vi "Error Message.vi"(8 "firmware revision":string(combo), 11 "error number":i32) -> (2 "error message":string)   [LabVIEW 2020, in "Andeen-Hagerling 2700A.lvlib"]
doc: "This VI returns takes an error number and returns a text error message. Firmware version is a parameter also because error messages differ across firmware versions."
uses:
  Andeen-Hagerling 2700A.lvlib
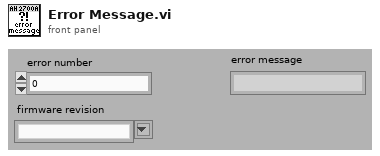
[diagram p1: front panel]
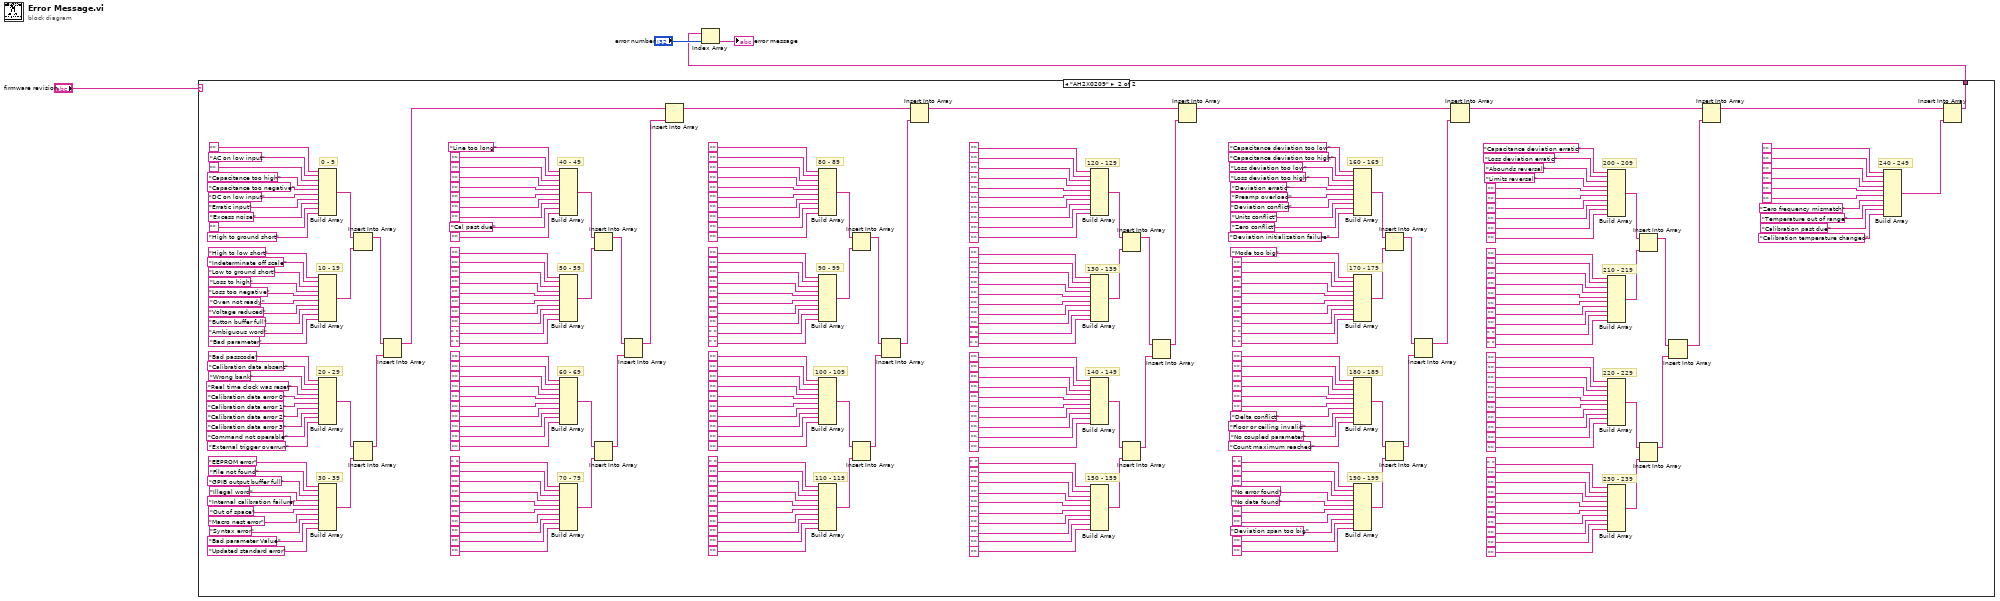
[diagram p0: block diagram]
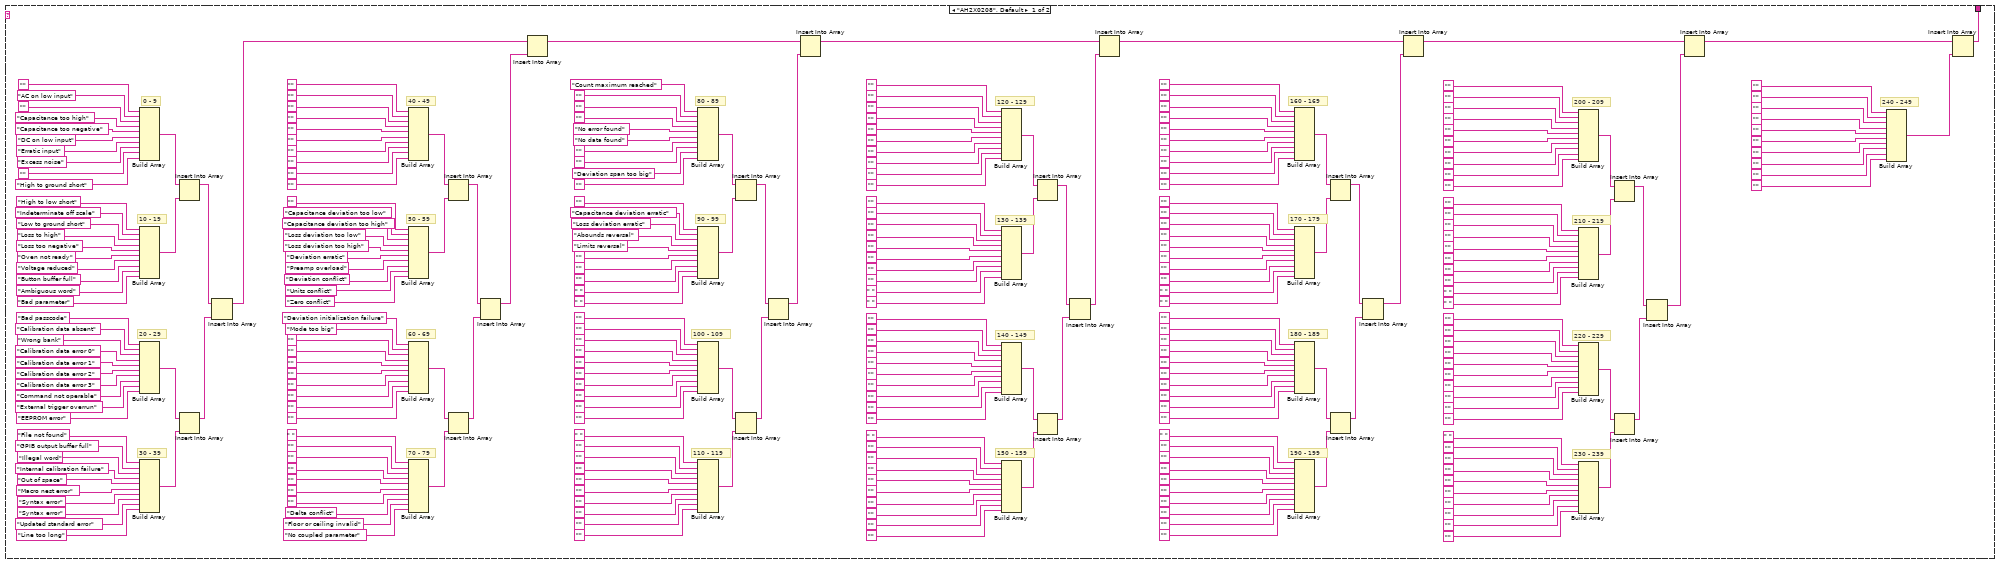
[diagram p2: hidden frame]
diagram:
  n1 = case shown="\"AH2X0209\"" "firmware revision" {
    tunnel: [w7 w304] -> w1
    frame "AH2X0208", Default {
      # "240 - 249"
      # "230 - 239"
      # "220 - 229"
      # "210 - 219"
      # "200 - 209"
      # "190 - 199"
      # "180 - 189"
      # "170 - 179"
      # "160 - 169"
      # "150 - 159"
      # "140 - 149"
      # "130 - 139"
      # "120 - 129"
      # "110 - 119"
      # "100 - 109"
      # "90 - 99"
      # "80 - 89"
      # "70 - 79"
      # "60 - 69"
      # "50 - 59"
      # "40 - 49"
      # "30 - 39"
      # "20 - 29"
      # "10 - 19"
      # "0 - 9"
      n2 = Build Array("", "AC on low input", "", "Capacitance too high", "Capacitance too negative", "DC on low input", "Erratic input", "Excess noise", "", "High to ground short") -> (w28:string[])
      n3 = Build Array("High to low short", "Indeterminate off scale", "Low to ground short", "Loss to high", "Loss too negative", "Oven not ready", "Voltage reduced", "Button buffer full", "Ambiguous word", "Bad parameter") -> (w29:string[])
      n4 = Build Array("Bad passcode", "Calibration data absent", "Wrong bank", "Calibration data error 0", "Calibration data error 1", "Calibration data error 2", "Calibration data error 3", "Command not operable", "External trigger overrun", "EEPROM error") -> (w40:string[])
      n5 = Build Array("File not found", "GPIB output buffer full", "Illegal word", "Internal calibration failure", "Out of space", "Macro nest error", "Syntax error", "Syntax error", "Updated standard error", "Line too long") -> (w41:string[])
      n6 = Insert Into Array(array=w28, new element=w29) -> (w52:string[])  [unwired: 1 in]
      n7 = Insert Into Array(array=w40, new element=w41) -> (w53:string[])  [unwired: 1 in]
      n8 = Insert Into Array(array=w52, new element=w53) -> (w292:string[])  [unwired: 1 in]
      n9 = Build Array("", "", "", "", "", "", "", "", "", "") -> (w72:string[])
      n10 = Build Array("", "Capacitance deviation too low", "Capacitance deviation too high", "Loss deviation too low", "Loss deviation too high", "Deviation erratic", "Preamp overload", "Deviation conflict", "Units conflict", "Zero conflict") -> (w73:string[])
      n11 = Build Array("Deviation initialization failure", "Mode too big", "", "", "", "", "", "", "", "") -> (w84:string[])
      n12 = Build Array(" ", "", "", "", "", "", "", "Delta conflict", "Floor or ceiling invalid", "No coupled parameter") -> (w85:string[])
      n13 = Insert Into Array(array=w72, new element=w73) -> (w96:string[])  [unwired: 1 in]
      n14 = Insert Into Array(array=w84, new element=w85) -> (w97:string[])  [unwired: 1 in]
      n15 = Insert Into Array(array=w96, new element=w97) -> (w293:string[])  [unwired: 1 in]
      n16 = Insert Into Array(array=w292, new element=w293) -> (w294:string[])  [unwired: 1 in]
      n17 = Build Array("Count maximum reached", "", "", "", "No error found", "No data found", "", "", "Deviation span too big", "") -> (w118:string[])
      n18 = Build Array("", "Capacitance deviation erratic", "Loss deviation erratic", "Abounds reversal", "Limits reversal", "", "", "", " ", " ") -> (w119:string[])
      n19 = Build Array("", "", "", "", "", "", "", "", "", "") -> (w130:string[])
      n20 = Build Array(" ", "", "", "", "", "", "", "", "", "") -> (w131:string[])
      n21 = Insert Into Array(array=w118, new element=w119) -> (w142:string[])  [unwired: 1 in]
      n22 = Insert Into Array(array=w130, new element=w131) -> (w143:string[])  [unwired: 1 in]
      n23 = Insert Into Array(array=w142, new element=w143) -> (w295:string[])  [unwired: 1 in]
      n24 = Insert Into Array(array=w294, new element=w295) -> (w296:string[])  [unwired: 1 in]
      n25 = Build Array("", "", "", "", "", "", "", "", "", "") -> (w164:string[])
      n26 = Build Array("", "", "", "", "", "", "", "", " ", " ") -> (w165:string[])
      n27 = Build Array("", "", "", "", "", "", "", "", "", "") -> (w176:string[])
      n28 = Build Array(" ", "", "", "", "", "", "", "", "", "") -> (w177:string[])
      n29 = Insert Into Array(array=w164, new element=w165) -> (w188:string[])  [unwired: 1 in]
      n30 = Insert Into Array(array=w176, new element=w177) -> (w189:string[])  [unwired: 1 in]
      n31 = Insert Into Array(array=w188, new element=w189) -> (w297:string[])  [unwired: 1 in]
      n32 = Insert Into Array(array=w296, new element=w297) -> (w298:string[])  [unwired: 1 in]
      n33 = Build Array("", "", "", "", "", "", "", "", "", "") -> (w210:string[])
      n34 = Build Array("", "", "", "", "", "", "", "", " ", " ") -> (w211:string[])
      n35 = Build Array("", "", "", "", "", "", "", "", "", "") -> (w222:string[])
      n36 = Build Array(" ", "", "", "", "", "", "", "", "", "") -> (w223:string[])
      n37 = Insert Into Array(array=w210, new element=w211) -> (w234:string[])  [unwired: 1 in]
      n38 = Insert Into Array(array=w222, new element=w223) -> (w235:string[])  [unwired: 1 in]
      n39 = Insert Into Array(array=w234, new element=w235) -> (w299:string[])  [unwired: 1 in]
      n40 = Insert Into Array(array=w298, new element=w299) -> (w300:string[])  [unwired: 1 in]
      n41 = Build Array("", "", "", "", "", "", "", "", "", "") -> (w256:string[])
      n42 = Build Array("", "", "", "", "", "", "", "", " ", " ") -> (w257:string[])
      n43 = Build Array("", "", "", "", "", "", "", "", "", "") -> (w268:string[])
      n44 = Build Array(" ", "", "", "", "", "", "", "", "", "") -> (w269:string[])
      n45 = Insert Into Array(array=w256, new element=w257) -> (w280:string[])  [unwired: 1 in]
      n46 = Insert Into Array(array=w268, new element=w269) -> (w281:string[])  [unwired: 1 in]
      n47 = Insert Into Array(array=w280, new element=w281) -> (w301:string[])  [unwired: 1 in]
      n48 = Insert Into Array(array=w300, new element=w301) -> (w302:string[])  [unwired: 1 in]
      n49 = Build Array("", "", "", "", "", "", "", "", "", "") -> (w303:string[])
      n50 = Insert Into Array(array=w302, new element=w303) -> (w7:string[])  [unwired: 1 in]
    }
    frame "AH2X0209" {
      # "240 - 249"
      # "230 - 239"
      # "220 - 229"
      # "210 - 219"
      # "200 - 209"
      # "190 - 199"
      # "180 - 189"
      # "170 - 179"
      # "160 - 169"
      # "150 - 159"
      # "140 - 149"
      # "130 - 139"
      # "120 - 129"
      # "110 - 119"
      # "100 - 109"
      # "90 - 99"
      # "80 - 89"
      # "70 - 79"
      # "60 - 69"
      # "50 - 59"
      # "40 - 49"
      # "30 - 39"
      # "20 - 29"
      # "10 - 19"
      # "0 - 9"
      n51 = Build Array("", "AC on low input", "", "Capacitance too high", "Capacitance too negative", "DC on low input", "Erratic input", "Excess noise", "", "High to ground short") -> (w325:string[])
      n52 = Build Array("High to low short", "Indeterminate off scale", "Low to ground short", "Loss to high", "Loss too negative", "Oven not ready", "Voltage reduced", "Button buffer full", "Ambiguous word", "Bad parameter") -> (w326:string[])
      n53 = Build Array("Bad passcode", "Calibration data absent", "Wrong bank", "Real time clock was reset", "Calibration data error 0", "Calibration data error 1", "Calibration data error 2", "Calibration data error 3", "Command not operable", "External trigger overrun") -> (w337:string[])
      n54 = Build Array("EEPROM error", "File not found", "GPIB output buffer full", "Illegal word", "Internal calibration failure", "Out of space", "Macro nest error", "Syntax error", "Bad parameter Value", "Updated standard error") -> (w338:string[])
      n55 = Insert Into Array(array=w325, new element=w326) -> (w349:string[])  [unwired: 1 in]
      n56 = Insert Into Array(array=w337, new element=w338) -> (w350:string[])  [unwired: 1 in]
      n57 = Insert Into Array(array=w349, new element=w350) -> (w591:string[])  [unwired: 1 in]
      n58 = Build Array("Line too long", "", "", "", "", "", "", "", "Cal past due", "") -> (w371:string[])
      n59 = Build Array("", "", "", "", "", "", "", "", " ", " ") -> (w372:string[])
      n60 = Build Array("", "", "", "", "", "", "", "", "", "") -> (w383:string[])
      n61 = Build Array(" ", "", "", "", "", "", "", "", "", "") -> (w384:string[])
      n62 = Insert Into Array(array=w371, new element=w372) -> (w395:string[])  [unwired: 1 in]
      n63 = Insert Into Array(array=w383, new element=w384) -> (w396:string[])  [unwired: 1 in]
      n64 = Insert Into Array(array=w395, new element=w396) -> (w592:string[])  [unwired: 1 in]
      n65 = Insert Into Array(array=w591, new element=w592) -> (w593:string[])  [unwired: 1 in]
      n66 = Build Array("", "", "", "", "", "", "", "", "", "") -> (w417:string[])
      n67 = Build Array("", "", "", "", "", "", "", "", " ", " ") -> (w418:string[])
      n68 = Build Array("", "", "", "", "", "", "", "", "", "") -> (w429:string[])
      n69 = Build Array(" ", "", "", "", "", "", "", "", "", "") -> (w430:string[])
      n70 = Insert Into Array(array=w417, new element=w418) -> (w441:string[])  [unwired: 1 in]
      n71 = Insert Into Array(array=w429, new element=w430) -> (w442:string[])  [unwired: 1 in]
      n72 = Insert Into Array(array=w441, new element=w442) -> (w594:string[])  [unwired: 1 in]
      n73 = Insert Into Array(array=w593, new element=w594) -> (w595:string[])  [unwired: 1 in]
      n74 = Build Array("", "", "", "", "", "", "", "", "", "") -> (w463:string[])
      n75 = Build Array("", "", "", "", "", "", "", "", " ", " ") -> (w464:string[])
      n76 = Build Array("", "", "", "", "", "", "", "", "", "") -> (w475:string[])
      n77 = Build Array(" ", "", "", "", "", "", "", "", "", "") -> (w476:string[])
      n78 = Insert Into Array(array=w463, new element=w464) -> (w487:string[])  [unwired: 1 in]
      n79 = Insert Into Array(array=w475, new element=w476) -> (w488:string[])  [unwired: 1 in]
      n80 = Insert Into Array(array=w487, new element=w488) -> (w596:string[])  [unwired: 1 in]
      n81 = Insert Into Array(array=w595, new element=w596) -> (w597:string[])  [unwired: 1 in]
      n82 = Build Array("Capacitance deviation too low", "Capacitance deviation too high", "Loss deviation too low", "Loss deviation too high", "Deviation erratic", "Preamp overload", "Deviation conflict", "Units conflict", "Zero conflict", "Deviation initialization failure") -> (w509:string[])
      n83 = Build Array("Mode too big", "", "", "", "", "", "", "", " ", " ") -> (w510:string[])
      n84 = Build Array("", "", "", "", "", "", "Delta conflict", "Floor or ceiling invalid", "No coupled parameter", "Count maximum reached") -> (w521:string[])
      n85 = Build Array(" ", "", "", "No error found", "No data found", "", "", "Deviation span too big", "", "") -> (w522:string[])
      n86 = Insert Into Array(array=w509, new element=w510) -> (w533:string[])  [unwired: 1 in]
      n87 = Insert Into Array(array=w521, new element=w522) -> (w534:string[])  [unwired: 1 in]
      n88 = Insert Into Array(array=w533, new element=w534) -> (w598:string[])  [unwired: 1 in]
      n89 = Insert Into Array(array=w597, new element=w598) -> (w599:string[])  [unwired: 1 in]
      n90 = Build Array("Capacitance deviation erratic", "Loss deviation erratic", "Abounds reversal", "Limits reversal", "", "", "", "", "", "") -> (w555:string[])
      n91 = Build Array("", "", "", "", "", "", "", "", " ", " ") -> (w556:string[])
      n92 = Build Array("", "", "", "", "", "", "", "", "", "") -> (w567:string[])
      n93 = Build Array(" ", "", "", "", "", "", "", "", "", "") -> (w568:string[])
      n94 = Insert Into Array(array=w555, new element=w556) -> (w579:string[])  [unwired: 1 in]
      n95 = Insert Into Array(array=w567, new element=w568) -> (w580:string[])  [unwired: 1 in]
      n96 = Insert Into Array(array=w579, new element=w580) -> (w600:string[])  [unwired: 1 in]
      n97 = Insert Into Array(array=w599, new element=w600) -> (w601:string[])  [unwired: 1 in]
      n98 = Build Array("", "", "", "", "", "", "Zero frequency mismatch", "Temperature out of range", "Calibration past due", "Calibration temperature changed") -> (w602:string[])
      n99 = Insert Into Array(array=w601, new element=w602) -> (w304:string[])  [unwired: 1 in]
    }
  }
  n100 = Index Array(array=w1, index="error number") -> (element=→"error message":string)
